vi "Check-client-activity.vi"(8 "error in (no error)":errorcluster, 9 "Check period":u32=5000 caption="Check period [ms]", 11 "ModComm in":T2) -> (0 "error out":errorcluster, 2 "Active clients":T1(array[cluster]), 3 "ModComm out":T2)   [LabVIEW 2013, in "SLMServer.lvlib" / "SLMServer.lvclass"]
uses:
  SLMServer.lvclass
  Object-reference.ctl
  SLMServer.lvclass/SLMServer.ctl
  Read Client IDs.vi
  Read Last contact.vi
  Read Heartbeat timeout.vi
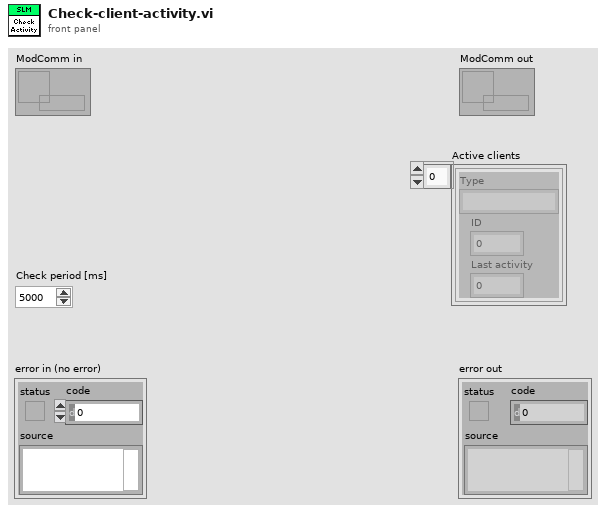
[diagram p1: front panel]
types:
  T1 = cluster{"Type":string, "ID":i32, "Last activity":i32}[]
  T2 = typedef "SLMServer.lvlib/SLMServer.lvclass/Object-reference.ctl" = refnum<data-value>
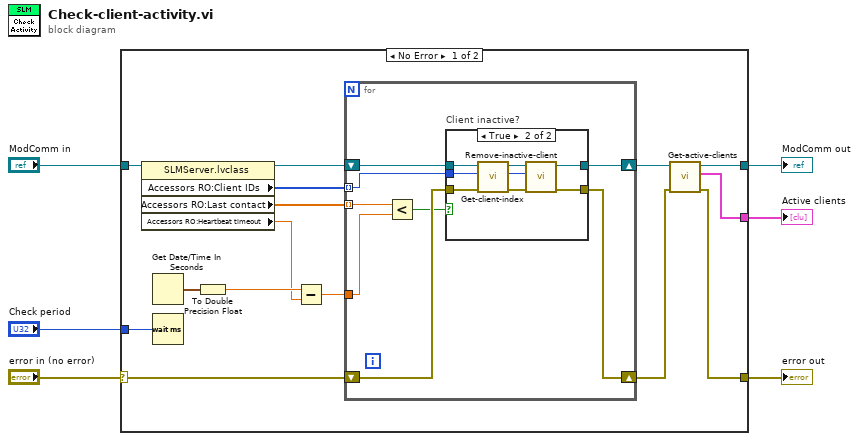
[diagram p0: block diagram]
diagram:
  n1 = case shown="No Error" "error in (no error)" {
    selector: "error in (no error)" -> [w12 w41]
    tunnel: [w8 w41] -> w5
    tunnel: [w10 w40] -> w3
    tunnel: "ModComm in" -> [w21 w40]
    tunnel: "Check period" -> [w20 _]
    tunnel: [w7 _] -> w1
    frame No Error {
      n2 = property class="SLMServer.lvclass"(reference=w21) -> (reference out=w13:T2, "Accessors RO:Client IDs"=w15:i32[], "Accessors RO:Last contact"=w16:dbl[], "Accessors RO:Heartbeat timeout"=w17:dbl)  [unwired: 1 in, 1 out]
      n3 = Get Date/Time In Seconds() -> (seconds since 1Jan1904=w19:timestamp)
      n4 = Wait (ms)(milliseconds to wait=w20) -> ()  [unwired: 1 out]
      n5 = To Double Precision Float(number=w19) -> (double precision float=w18:dbl)
      n6 = Subtract(x=w18, y=w17) -> (x-y=w14:dbl)
      n7 = for {
        tunnel: w16 -> [w29] mode=indexing
        tunnel: w15 -> [w22] mode=indexing
        tunnel: w14 -> [w28]
        shift-right: [w26] -> w11
        shift-left: w13 -> [w27]
        shift-right: [w24] -> w9
        shift-left: w12 -> [w25]
        n8 = Less?(x=w29, y=w28) -> (x < y?=w23:bool)
        n9 = case "Client inactive?" shown="True" w23 {
          tunnel: w27 -> [w31 w37]
          tunnel: [w31 w39] -> w26
          tunnel: w25 -> [w30 w33]
          tunnel: [w30 w38] -> w24
          tunnel: w22 -> [_ w34]
          frame False {
          }
          frame True {
            n10 = call "Get-client-index.vi"("error in (no error)"=w33, "Client ID"=w34, "ModComm in"=w37) -> ("error out"=w32:errorcluster, "Client index"=w35:i32, "ModComm out"=w36:T2)  [unwired: 6 in]
            n11 = call "Remove-inactive-client.vi"("error in (no error)"=w32, "Client index"=w35, "ModComm in"=w36) -> ("error out"=w38:errorcluster, "ModComm out"=w39:T2)  [unwired: 7 in]
          }
        }
      }
      n12 = call "Get-active-clients.vi"("error in (no error)"=w9, "ModComm in"=w11) -> ("error out"=w8:errorcluster, "Active clients"=w7:T1, "ModComm out"=w10:T2)  [unwired: 7 in]
    }
    frame Error {
    }
  }
  "error out" <- w5
  "ModComm out" <- w3
  "Active clients" <- w1
